vi "Enter IPs.vi"(9 "34972A IP":string="192.168.25.2", 10 "MW100 IP":string="192.168.25.4") -> (1 "34972A IP Out":string="192.168.25.2", 2 "MW100 IP Out":string="192.168.25.4")   [LabVIEW 2012]
panel:
  in  "Enter IPs":bool
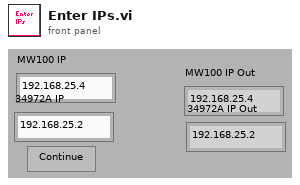
[diagram p1: front panel]
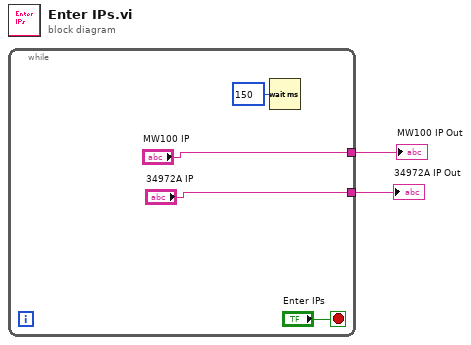
[diagram p0: block diagram]
diagram:
  n1 = while {
    tunnel: ["MW100 IP"] -> w2
    tunnel: ["34972A IP"] -> w1
    stop <- "Enter IPs" stop-if-true
    n2 = Wait (ms)(milliseconds to wait=u32 150) -> ()  [unwired: 1 out]
  }
  "MW100 IP Out" <- w2
  "34972A IP Out" <- w1
